vi "Chloe's Furnace.vi"() -> ()   [LabVIEW 2013]
panel:
  in  "Thermometer":dbl(slide) scale=0.0..100.0
  out "Boolean":bool caption="Furnace Switch"
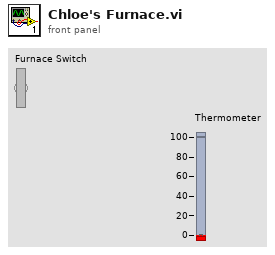
[diagram p1: front panel]
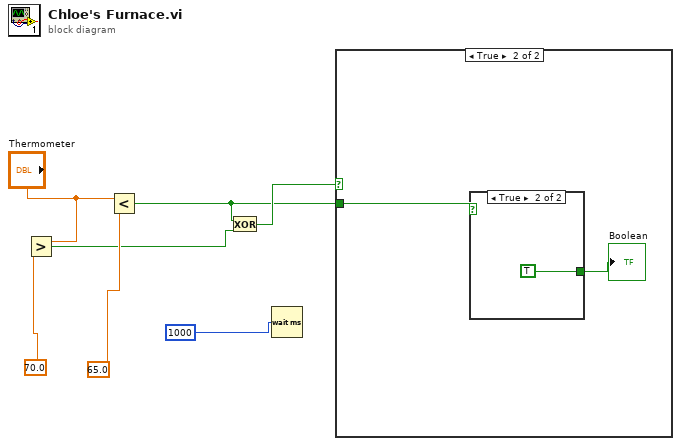
[diagram p0: block diagram]
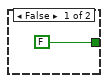
[diagram p3: hidden frame]
diagram:
  n1 = Greater?(x="Thermometer", y=70.0) -> (0:w4:bool)
  n2 = Less?(x="Thermometer", y=65.0) -> (x < y?=w2:bool)
  n3 = Exclusive Or(1:w4, 2:w2) -> (0:w3:bool)
  n4 = Wait (ms)(milliseconds to wait=u32 1000 ("millisecond timer value")) -> ()  [unwired: 1 out]
  n5 = case shown="True" w3 {
    tunnel: w2 -> [_ w9]
    frame False {
    }
    frame True {
      n6 = case shown="True" w9 {
        tunnel: [FALSE TRUE] -> w8
        frame False {
        }
        frame True {
        }
      }
      "Boolean" <- w8
    }
  }
